vi "resetOutput.vi"(8 "error in (no error)":errorcluster, 11 "niDAQmxAO in":refnum<class "niDAQmxAO.lvclass">) -> (0 "error out":errorcluster, 3 "niDAQmxAO out":refnum<class "niDAQmxAO.lvclass">)   [LabVIEW 2009, in "Hardware.lvlib" / "Channels.lvlib" / "niDAQmxAO.lvclass"]
uses:
  niDAQmxAO.lvclass
  <vilib>/DAQmx/write.llb/DAQmx Write (Analog 1D DBL NChan 1Samp).vi
  <vilib>/DAQmx/create/channels.llb/DAQmx Create Channel (AO-Voltage-Basic).vi
  AnalogOutput.lvclass
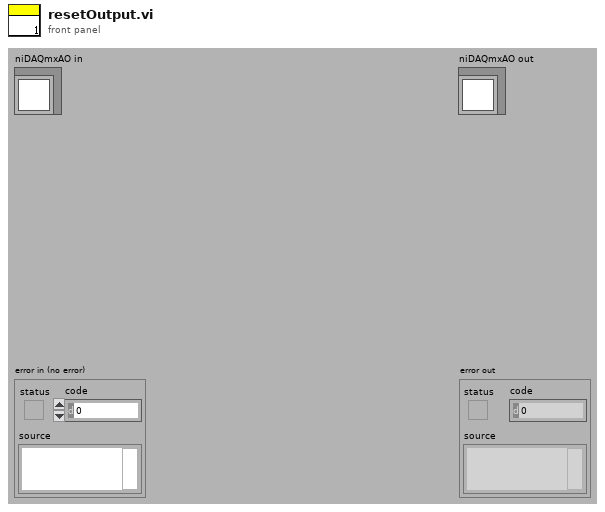
[diagram p1: front panel]
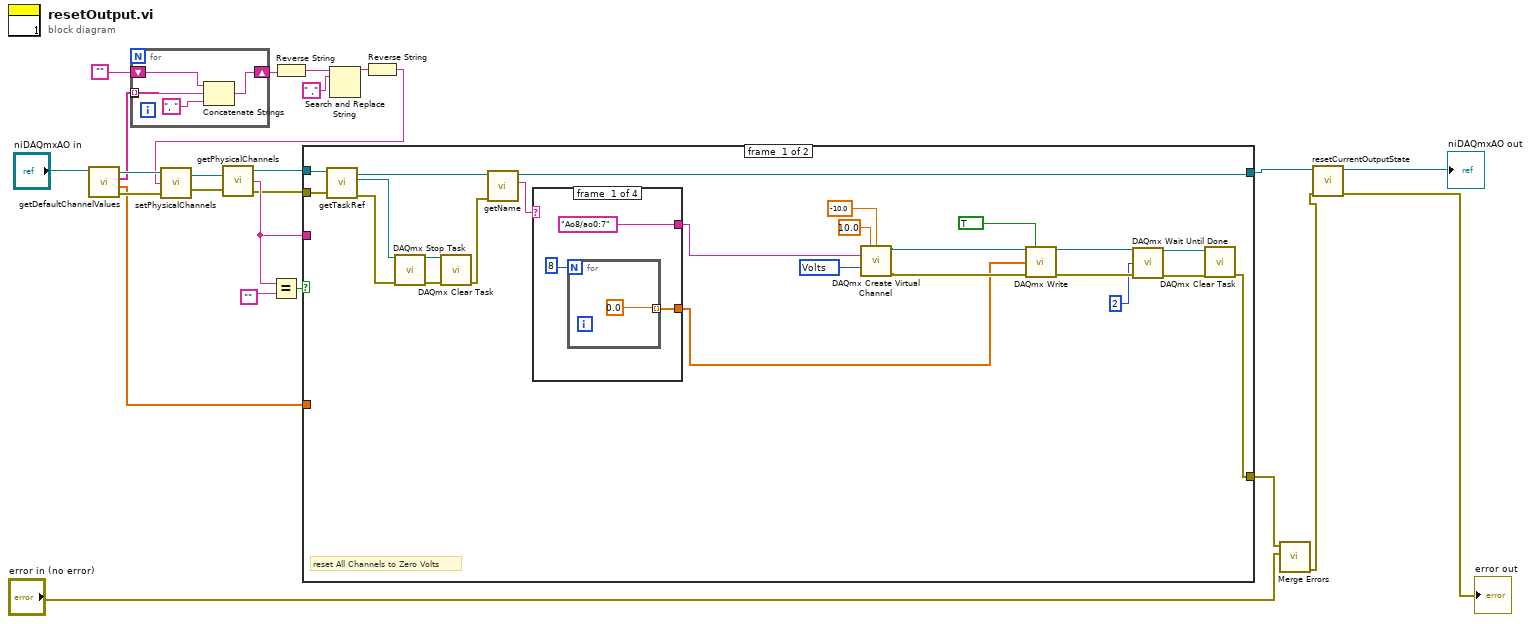
[diagram p0: block diagram]
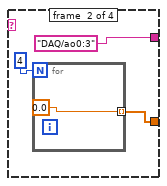
[diagram p2: hidden frame]
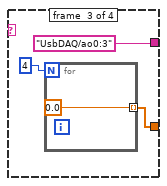
[diagram p3: hidden frame]
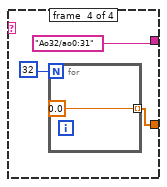
[diagram p4: hidden frame]
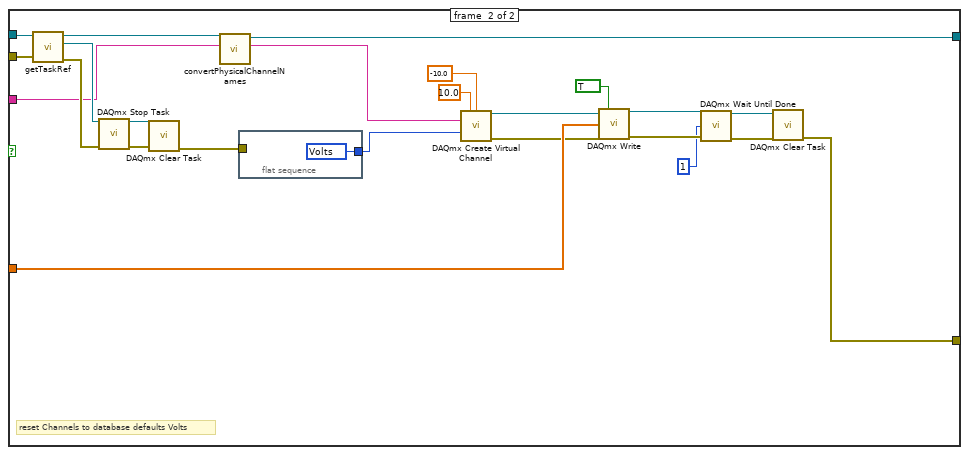
[diagram p5: hidden frame]
diagram:
  n1 = call "getDefaultChannelValues.vi"("AnalogOutput in"="niDAQmxAO in") -> ("error out"=w6:errorcluster, "calibratedValues"=w5:dbl[], "channel_addresses"=w13:string[], "AnalogOutput out"=w16:refnum<class "niDAQmxAO.lvclass">)  [unwired: 7 in]
  n2 = for {
    tunnel: [w27] -> _ mode=indexing
    tunnel: w13 -> [w27] mode=indexing
    shift-right: [w25] -> w11
    shift-left: "" -> [w28]
    n3 = Concatenate Strings(w28, w27, ", ") -> (w25:string)
  }
  n4 = Reverse String(1:w11) -> (0:w10:string)
  n5 = Search and Replace String(input string=w10, search string=" ,") -> (result string=w8:string)  [unwired: 6 in, 3 out]
  n6 = Reverse String(1:w8) -> (0:w7:string)
  n7 = call-dynamic "setPhysicalChannels.vi"("error in (no error)"=w6, "Physical Channels"=w7, "AnalogOutput.lvclass in"=w16) -> ("error out"=w14:errorcluster, "AnalogOutput.lvclass out"=w15:refnum<class "niDAQmxAO.lvclass">)
  n8 = call-dynamic "getPhysicalChannels.vi"("AnalogOutput.lvclass in"=w15, "error in (no error)"=w14) -> ("AnalogOutput.lvclass out"=w21:refnum<class "niDAQmxAO.lvclass">, "Physical Channels"=w22:string, "error out"=w20:errorcluster)
  n9 = Equal?(x=w22, y="") -> (x = y?=w23:bool)
  n10 = case shown="False" w23 {
    tunnel: w22 -> [_ w75]
    tunnel: w21 -> [w52 w92]
    tunnel: [w44 w73] -> w4
    tunnel: w20 -> [w51 w91]
    tunnel: [w37 w81] -> w19
    tunnel: w5 -> [_ w71]
    frame #0 {
      w29 = 10348 items=["Volts"=10348, "From Custom Scale"=10065] ("units")
      # "reset All Channels to Zero Volts"
      n11 = call "getTaskRef.vi"("error in (no error)"=w51, "niDAQmxAO.lvclass in"=w52) -> ("error out"=w49:errorcluster, "DAQmx Task Ref"=w50:refnum<k21>, "niDAQmxAO.lvclass out"=w46:refnum<class "niDAQmxAO.lvclass">)  [unwired: 7 in]
      n12 = call <vilib>:"DAQmx Stop Task.vi"("task/channels in"=w50, "error in"=w49) -> ("task out"=w48:refnum<k21>, "error out"=w47:errorcluster)  [unwired: 12 in]
      n13 = call <vilib>:"DAQmx Clear Task.vi"("task in"=w48, "error in"=w47) -> ("error out"=w45:errorcluster)  [unwired: 13 in]
      n14 = call "getName.vi"("error in (no error)"=w45, "AnalogOutput.lvclass in"=w46) -> ("name"=w43:string, "AnalogOutput.lvclass out"=w44:refnum<class "niDAQmxAO.lvclass">)  [unwired: 7 in, 1 out]
      n15 = case shown="\"Ao8\", Default" w43 {
        tunnel: ["Ao8/ao0:7" "DAQ/ao0:3" "UsbDAQ/ao0:3" "Ao32/ao0:31"] -> w30
        tunnel: [w53 w57 w61 w65] -> w31
        frame #0 {
          n16 = for {
            N: 8 -> [_]
            tunnel: [0.0] -> w53 mode=indexing
          }
        }
        frame #1 {
          n17 = for {
            N: 4 -> [_]
            tunnel: [0.0] -> w57 mode=indexing
          }
        }
        frame #2 {
          n18 = for {
            N: 4 -> [_]
            tunnel: [0.0] -> w61 mode=indexing
          }
        }
        frame #3 {
          n19 = for {
            N: 32 -> [_]
            tunnel: [0.0] -> w65 mode=indexing
          }
        }
      }
      n20 = call-poly <vilib>:"DAQmx Create Virtual Channel.vi"("maximum value"=10.0, "minimum value"=-10.0, "physical channels"=w30, "units"=w29) -> ("task out"=w33:refnum<k21>, "error out"=w32:errorcluster)  [unwired: 10 in]
      n21 = call-poly <vilib>:"DAQmx Write.vi"("task/channels in"=w33, "auto start"=TRUE, "data"=w31, "error in"=w32) -> ("task out"=w41:refnum<k21>, "error out"=w40:errorcluster)  [unwired: 9 in, 1 out]
      n22 = call <vilib>:"DAQmx Wait Until Done.vi"("task/channels in"=w41, "timeout (sec)"=2, "error in"=w40) -> ("task out"=w39:refnum<k21>, "error out"=w38:errorcluster)  [unwired: 11 in]
      n23 = call <vilib>:"DAQmx Clear Task.vi"("task in"=w39, "error in"=w38) -> ("error out"=w37:errorcluster)  [unwired: 13 in]
    }
    frame #1 {
      # "reset Channels to database defaults Volts"
      n24 = call "getTaskRef.vi"("error in (no error)"=w91, "niDAQmxAO.lvclass in"=w92) -> ("error out"=w89:errorcluster, "DAQmx Task Ref"=w90:refnum<k21>, "niDAQmxAO.lvclass out"=w74:refnum<class "niDAQmxAO.lvclass">)  [unwired: 7 in]
      n25 = call <vilib>:"DAQmx Stop Task.vi"("task/channels in"=w90, "error in"=w89) -> ("task out"=w80:refnum<k21>, "error out"=w79:errorcluster)  [unwired: 12 in]
      n26 = call <vilib>:"DAQmx Clear Task.vi"("task in"=w80, "error in"=w79) -> ("error out"=w78:errorcluster)  [unwired: 13 in]
      n27 = call "convertPhysicalChannelNames.vi"("PhysicalChannels"=w75, "niDAQmxAO.lvclass in"=w74) -> ("channel_names"=w72:string, "niDAQmxAO.lvclass out"=w73:refnum<class "niDAQmxAO.lvclass">)  [unwired: 7 in, 1 out]
      n28 = flat-sequence {
        tunnel: w78 -> [_]
        tunnel: [w93] -> w77
        frame #0 {
          w93 = 10348 items=["Volts"=10348, "From Custom Scale"=10065] ("units")
        }
      }
      n29 = call-poly <vilib>:"DAQmx Create Virtual Channel.vi"("maximum value"=10.0, "minimum value"=-10.0, "physical channels"=w72, "units"=w77) -> ("task out"=w70:refnum<k21>, "error out"=w69:errorcluster)  [unwired: 10 in]
      n30 = call-poly <vilib>:"DAQmx Write.vi"("task/channels in"=w70, "auto start"=TRUE, "data"=w71, "error in"=w69) -> ("task out"=w85:refnum<k21>, "error out"=w84:errorcluster)  [unwired: 9 in, 1 out]
      n31 = call <vilib>:"DAQmx Wait Until Done.vi"("task/channels in"=w85, "timeout (sec)"=1, "error in"=w84) -> ("task out"=w83:refnum<k21>, "error out"=w82:errorcluster)  [unwired: 11 in]
      n32 = call <vilib>:"DAQmx Clear Task.vi"("task in"=w83, "error in"=w82) -> ("error out"=w81:errorcluster)  [unwired: 13 in]
    }
  }
  n33 = call <vilib>:"Merge Errors.vi"("error in 2 (no error)"="error in (no error)", "error in 1 (no error)"=w19) -> ("error out"=w2:errorcluster)  [unwired: 5 in]
  n34 = call "resetCurrentOutputState.vi"("error in (no error)"=w2, "AnalogOutput in"=w4) -> ("error out"=→"error out":errorcluster, "AnalogOutput out"=→"niDAQmxAO out":refnum<class "niDAQmxAO.lvclass">)  [unwired: 8 in]
